vi "SUB_FindSpecific_OriginalString.vi"(3 "Find this String":string, 5 "String data":string) -> (0 "before \"; \" string":string, 2 "Found":bool)   [LabVIEW 2011]
panel:
  out "after substring":string
  out "match substring":string
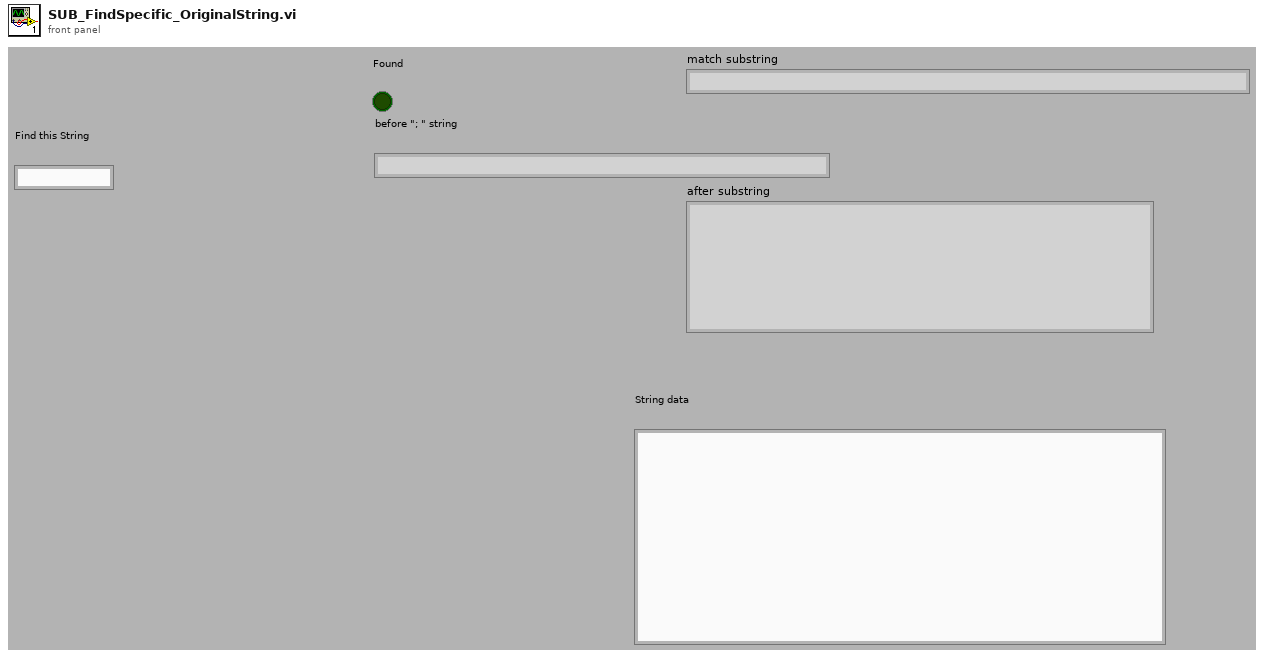
[diagram p1: front panel]
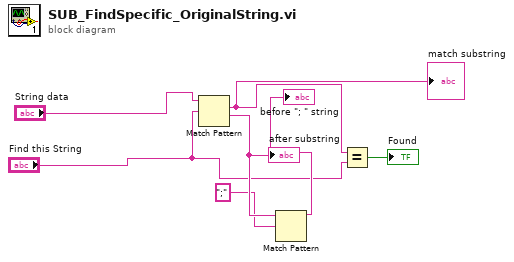
[diagram p0: block diagram]
diagram:
  n1 = Match Pattern(string="String data", regular expression="Find this String") -> (match substring=w5:string, after substring=w7:string)  [unwired: 1 in, 2 out]
  "match substring" <- w5
  "after substring" <- w7
  n2 = Match Pattern(string=w7, regular expression=";") -> (before substring=→"before \"; \" string":string)  [unwired: 1 in, 3 out]
  n3 = Equal?(x=w5, y="Find this String") -> (x = y?=→"Found":bool)
